vi "NMR14.vi"() -> ()   [LabVIEW 2013]
uses:
  <vilib>/Utility/file.llb/Read From Spreadsheet File (DBL).vi
  <vilib>/Analysis/NI_AALBase.lvlib
panel:
  in  "Q curve file":string="realback213.txt"
  out "File name 2":string="C:\\users\\plm\\Desktop\\rssmt\\realback213.txt"
  in  "AutoBaseline":bool
  out "RF OK":bool=TRUE
  out "Peak area (V-MHz)":sgl=3.3948524 format="%.3f"
  in  "Gauss Fit":bool
  out "NMR Graph + Fit":cluster{cluster{dbl, "Numeric":dbl}[]}[](graph)=[{[{212.6, "Numeric"=6.179833984375}, {212.608, "Numeric"=5.96031494140625}, {212.61599999999999, "Numeric"=5.74044189453125}, {212.624, "Numeric"=5.5264892578125}, {212.632, "Numeric"=5.31328125}, {212.64, "Numeric"=5.10472412109375}, {212.648, "Numeric"=4.900927734375}, {212.656, "Numeric"=4.704541015625}, {212.664, "Numeric"=4.511669921875}, {212.672, "Numeric"=4.3124755859375}, {212.68, "Numeric"=4.1198974609375}, {212.688, "Numeric"=3.935693359375}, {212.696, "Numeric"=3.76107177734375}, {212.704, "Numeric"=3.5800537109375}, {212.712, "Numeric"=3.40418701171875}, {212.72, "Numeric"=3.2398681640625}, {212.728, "Numeric"=3.0807373046875}, {212.736, "Numeric"=2.91600341796875}, {212.744, "Numeric"=2.76717529296875}, {212.752, "Numeric"=2.60875244140625}, {212.76, "Numeric"=2.45557861328125}, {212.768, "Numeric"=2.3186279296875}, {212.776, "Numeric"=2.17218017578125}, {212.784, "Numeric"=2.04324951171875}, {212.792, "Numeric"=1.9197265625}, {212.79999999999998, "Numeric"=1.78963623046875}, {212.808, "Numeric"=1.67039794921875}, {212.816, "Numeric"=1.54791259765625}, {212.82399999999998, "Numeric"=1.44422607421875}, {212.832, "Numeric"=1.32734375}, {212.84, "Numeric"=1.22919921875}, {212.84799999999998, "Numeric"=1.13302001953125}, {212.856, "Numeric"=1.03822021484375}, {212.864, "Numeric"=0.9540771484375}, {212.87199999999999, "Numeric"=0.87376708984375}, {212.88, "Numeric"=0.78779296875}, {212.888, "Numeric"=0.71485595703125}, {212.896, "Numeric"=0.63963623046875}, {212.904, "Numeric"=0.59088134765625}, {212.912, "Numeric"=0.532666015625}, {212.92, "Numeric"=0.4708251953125}, {212.928, "Numeric"=0.423828125}, {212.936, "Numeric"=0.37716064453125}, {212.944, "Numeric"=0.3446533203125}, {212.952, "Numeric"=0.32086181640625}, {212.96, "Numeric"=0.2843017578125}, {212.968, "Numeric"=0.270751953125}, {212.976, "Numeric"=0.2579833984375}, {212.984, "Numeric"=0.23699951171875}, {212.992, "Numeric"=0.23897705078125}, {213.0, "Numeric"=0.238916015625}, {213.008, "Numeric"=0.248974609375}, {213.016, "Numeric"=0.265283203125}, {213.024, "Numeric"=0.28079833984375}, {213.032, "Numeric"=0.300244140625}, {213.04, "Numeric"=0.33636474609375}, {213.048, "Numeric"=0.372314453125}, {213.056, "Numeric"=0.4180908203125}, {213.064, "Numeric"=0.4687255859375}, {213.072, "Numeric"=0.525830078125}, {213.08, "Numeric"=0.58543701171875}, {213.088, "Numeric"=0.6470947265625}, {213.096, "Numeric"=0.7219970703125}, {213.104, "Numeric"=0.81129150390625}, {213.112, "Numeric"=0.90042724609375}, {213.12, "Numeric"=0.9976318359375}, {213.12800000000001, "Numeric"=1.0961669921875}, {213.136, "Numeric"=1.19154052734375}, {213.144, "Numeric"=1.30576171875}, {213.15200000000002, "Numeric"=1.42882080078125}, {213.16, "Numeric"=1.55714111328125}, {213.168, "Numeric"=1.69908447265625}, {213.17600000000002, "Numeric"=1.83853759765625}, {213.184, "Numeric"=1.98814697265625}, {213.192, "Numeric"=2.1465087890625}, {213.2, "Numeric"=2.30396728515625}, {213.208, "Numeric"=2.4755859375}, {213.216, "Numeric"=2.64779052734375}, {213.224, "Numeric"=2.8399658203125}, {213.232, "Numeric"=3.03016357421875}, {213.24, "Numeric"=3.2257568359375}, {213.248, "Numeric"=3.4392822265625}, {213.256, "Numeric"=3.6543701171875}, {213.264, "Numeric"=3.87130126953125}, {213.272, "Numeric"=4.10189208984375}, {213.28, "Numeric"=4.33153076171875}, {213.288, "Numeric"=4.5672119140625}, {213.296, "Numeric"=4.82923583984375}, {213.304, "Numeric"=5.08277587890625}, {213.312, "Numeric"=5.3467041015625}, {213.32, "Numeric"=5.62410888671875}, {213.328, "Numeric"=5.90218505859375}, {213.336, "Numeric"=6.19228515625}, {213.344, "Numeric"=6.49820556640625}, {213.352, "Numeric"=6.7964599609375}, {213.36, "Numeric"=7.11771240234375}, {213.368, "Numeric"=7.44090576171875}, {213.376, "Numeric"=7.7695068359375}, {213.38400000000001, "Numeric"=8.12364501953125}, {213.392, "Numeric"=8.476611328125}, {213.4, "Numeric"=8.8313720703125}]}]
  in  "Amp of Q curve":dbl=1.7999999999999998 min=0.0 max=3.0 step=0.01 format="%_3f"
  in  "Subtract Q curve":bool
  in  "Adjust Tune":bool
  out "IF Offset":dbl(graph)=1.8102946533203148
  out "Pedestal Difference":dbl(graph)=1.261193033854167
  out "# Good Spectra":i32=1
  in  "Quality cuts":bool=TRUE
  out "Pedestal OK":bool
  out "Sweep #":i32=100
  out "1st Sweep":bool
  out "ADC volts OK":bool=TRUE
  out "Peak Height Distribution":cluster{"Y":dbl[], "Y":dbl[]}[](graph)=[{"Y"=[-99.0, -99.0, -99.0, -99.0, -99.0, -99.0, -99.0, -99.0, -99.0, -99.0, -99.0, -99.0, -99.0, -99.0, -99.0, -99.0, -99.0, -99.0, -99.0, -99.0, -99.0, -99.0, -99.0, -99.0, -99.0, -99.0, -99.0, -99.0, -99.0, -99.0, -99.0, -99.0, -99.0, -99.0, -99.0, -99.0, -99.0, -99.0, -99.0, -99.0, -99.0, -99.0, -99.0, -99.0, -99.0, -99.0, -99.0, -99.0, -99.0, -99.0, -99.0, -99.0, -99.0, -99.0, -99.0, -99.0, -99.0, -99.0, -99.0, -99.0, -99.0, -99.0, -99.0, -99.0, -99.0, -99.0, -99.0, -99.0, -99.0, -99.0, -99.0, -99.0, -99.0, -99.0, -99.0, -99.0, -99.0, -99.0, -99.0, -99.0, -99.0, -99.0, -99.0, -99.0, -99.0, -99.0, -99.0, -99.0, -99.0, -99.0, -99.0, -99.0, -99.0, -99.0, -99.0, -99.0, -99.0, -99.0, -99.0, -99.0], "Y"=[0.0, 0.0, 0.0, 0.0, 0.0, 0.0, 0.0, 0.0, 0.0, 0.0, 0.0, 0.0, 0.0, 0.0, 0.0, 0.0, 0.0, 0.0, 0.0, 0.0, 0.0, 0.0, 0.0, 0.0, 0.0, 0.0, 0.0, 0.0, 0.0, 0.0, 0.0, 0.0, 0.0, 0.0, 0.0, 0.0, 0.0, 0.0, 0.0, 0.0, 0.0, 0.0, 0.0, 0.0, 0.0, 0.0, 0.0, 0.0, 0.0, 0.0, 0.0, 0.0, 0.0, 0.0, 0.0, 0.0, 0.0, 0.0, 0.0, 0.0, 0.0, 0.0, 0.0, 0.0, 0.0, 0.0, 0.0, 0.0, 0.0, 0.0, 0.0, 0.0, 0.0, 0.0, 0.0, 0.0, 0.0, 0.0, 0.0, 0.0, 0.0, 0.0, 0.0, 0.0, 0.0, 0.0, 0.0, 0.0, 0.0, 0.0, 0.0, 0.0, 0.0, 0.0, 0.0, 0.0, 0.0, 0.0, 0.0, 1.0]}]
  in  "# of Sweeps":i32=100
  out "Std Dev (V)":dbl=nan format="%_2g"
  out "Peak mean (V)":dbl=-99.0 format="%_4g"
  out "Peak Height":dbl(graph)=8.8313720703125
  in  "Raw Data":bool=TRUE
  in  "Tank RF ON":bool=TRUE
  in  "IF Atten (dB)":i8 min=0 max=35 step=5
  in  "IFoffset (V)":dbl=1.8102946533203148 min=0.0 max=3000.0 step=0.001 format="%.3f"
  in  "Tune  (V)":dbl=1.6310000000000064 min=0.0 max=5.0 step=0.001 format="%.3f"
  in  "Hi / Lo Gain":bool
  out "Voltage Array":sgl[](array[numeric])=[6.179834, 5.9603148, 5.740442, 5.5264893, 5.313281, 5.104724, 4.9009275, 4.704541, 4.51167, 4.3124757, 4.1198974, 3.9356933, 3.7610717, 3.5800538, 3.404187, 3.2398682, 3.0807374, 2.9160035, 2.7671752, 2.6087525, 2.4555786, 2.3186278, 2.1721802, 2.0432496, 1.9197266, 1.7896363, 1.670398, 1.5479126, 1.444226, 1.3273437, 1.2291992, 1.13302, 1.0382202, 0.9540771, 0.8737671, 0.787793, 0.71485597, 0.6396362, 0.59088135, 0.532666, 0.4708252, 0.42382812, 0.37716064, 0.3446533, 0.32086182, 0.28430176, 0.27075195, 0.2579834, 0.23699951, 0.23897704, 0.23891601, 0.2489746, 0.2652832, 0.28079835, 0.30024415, 0.33636475, 0.37231445, 0.41809082, 0.4687256, 0.5258301, 0.585437, 0.6470947, 0.7219971, 0.8112915, 0.9004272, 0.99763185, 1.096167, 1.1915405, 1.3057617, 1.4288208, 1.5571411, 1.6990845, 1.8385376, 1.988147, 2.1465087, 2.3039672, 2.475586, 2.6477904, 2.8399658, 3.0301635, 3.225757, 3.4392822, 3.65437, 3.8713012, 4.101892, 4.3315306, 4.567212, 4.829236, 5.082776, 5.346704, 5.624109, 5.902185, 6.192285, 6.4982057, 6.79646, 7.1177125, 7.4409056, 7.769507, 8.123645, 8.476611, 8.831372] format="%.4f"
  in  "Invert Polarity":bool=TRUE
  out "Pedestal Diff (V)":sgl=1.261193 format="%.3f"
  out "Peak amp (V)":sgl=8.831372 format="%.3f"
  in  "Save Data to File":bool=TRUE
  in  "RF Level (dBm)":dbl=-1.0 min=-10.0 max=1.0 step=0.1 format="%.2f"
  out "SMT error out":errorcluster
  out "Sample RMS (V)":dbl=0.008836833866740928 format="%.4f"
  in  "# Sample/step":i32=100 min=1 max=1000 step=100
  in  "ADC Rate (Hz)":i32=10000 min=1 max=20000 step=1000
  in  "ADC Range":i32(ring)=1 items=["+- 10 V"=1, "+- 2.5 V"=3]
  in  "Step Width (MHz)":dbl=0.008 min=0.0 max=1000.0 step=0.0005 format="%.4f"
  in  "Freq Span (MHz)":dbl=0.8 min=0.0 max=3000.0 step=0.1 format="%.3f"
  in  "Center Freq (MHz)":dbl=213.0 min=0.005 max=6000.0 step=0.1 format="%.3f"
  in  "Sweep Mode":u16(ring)=3 items=["Off", "Single", "Auto", "Step"]
  in  "GPIB Addr (28)":refnum<visa-resource-name>="GPIB0::28::INSTR"
  # "Settings"
  # "E1039 Prototype NMR Control Panel"
  # "D\nA\nC"
  # "R\nF\n\nG\ne\nn\ne\nr\na\nt\no\nr"
  # "A\nD\nC"
  # "D\na\nt\na"
  # "I\n/\nO"
  # "Results"
  # "A\nv\ne\nr\na\ng\ne"
  # "S\nw\ne\ne\np"
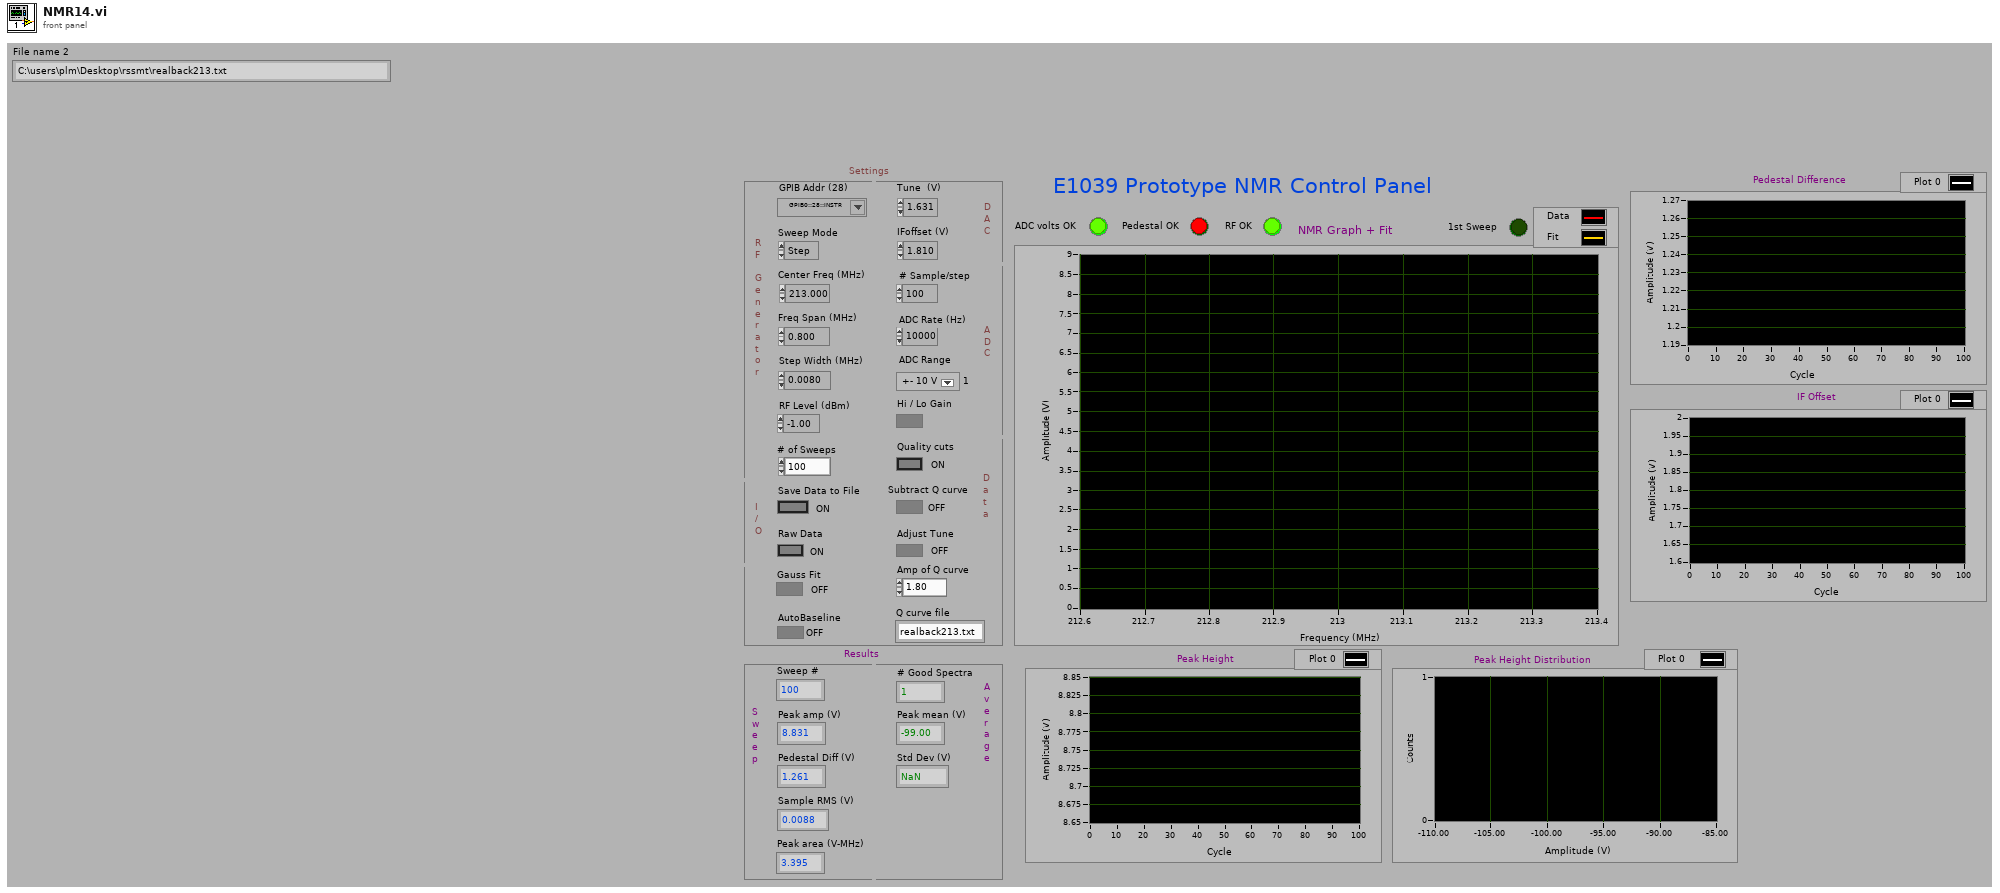
[diagram p1: front panel]
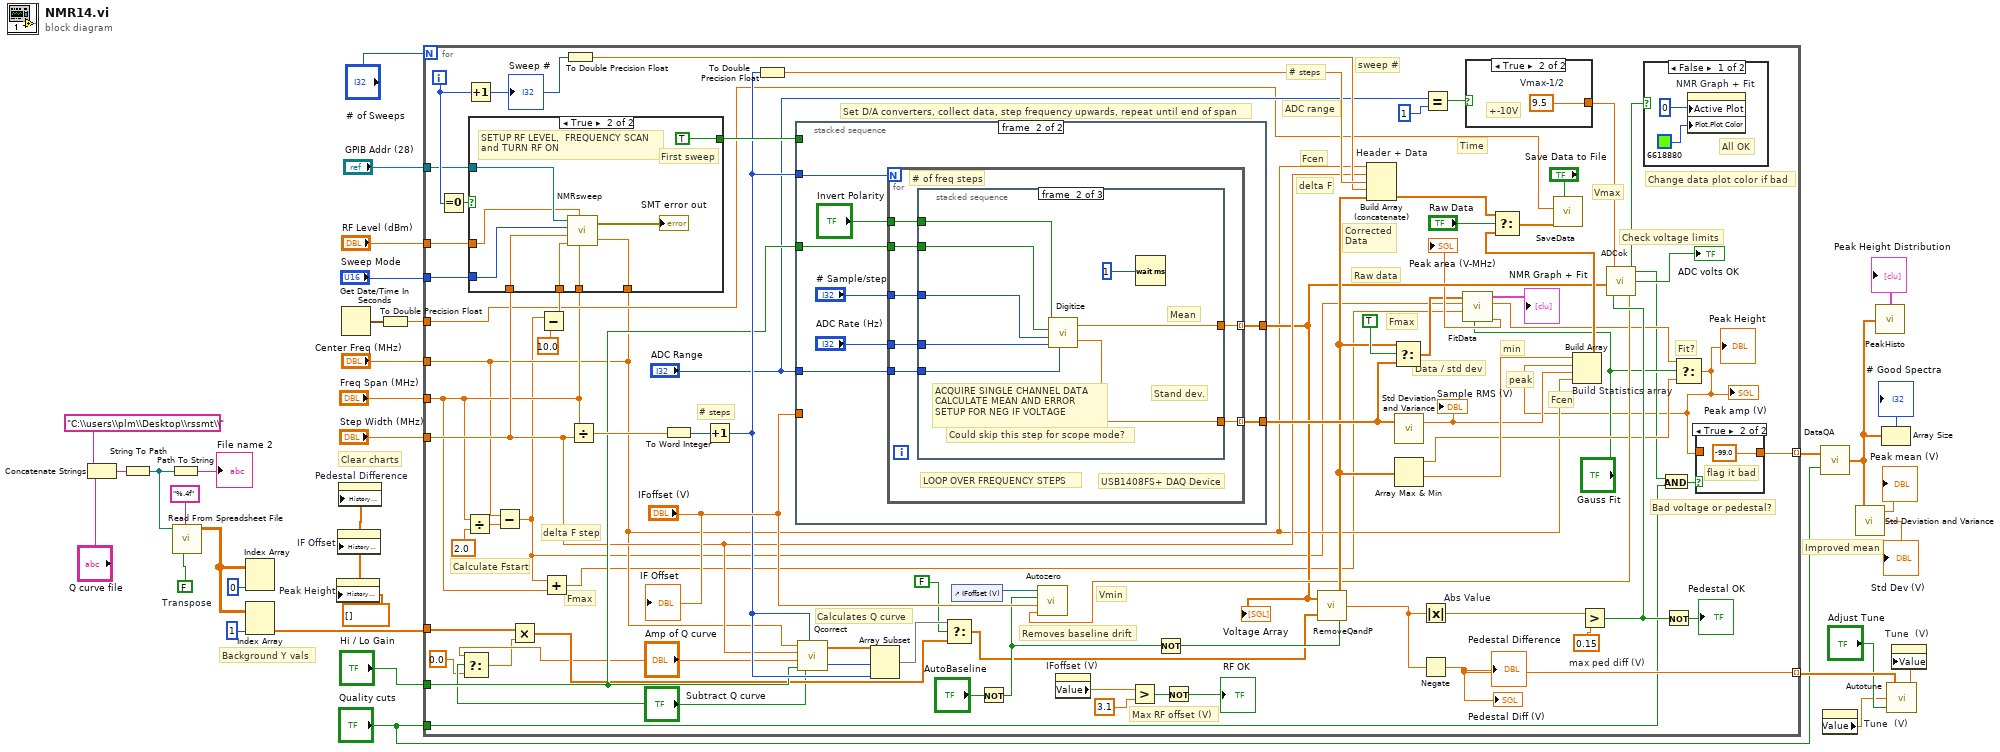
[diagram p0: block diagram]
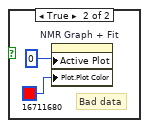
[diagram p2: hidden frame]
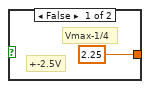
[diagram p3: hidden frame]
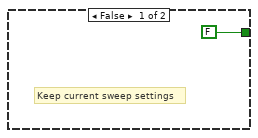
[diagram p5: hidden frame]
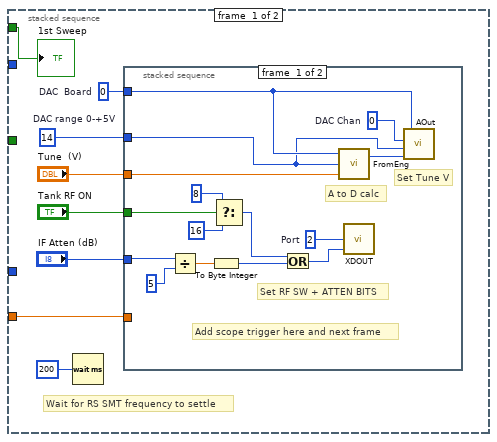
[diagram p6: hidden frame]
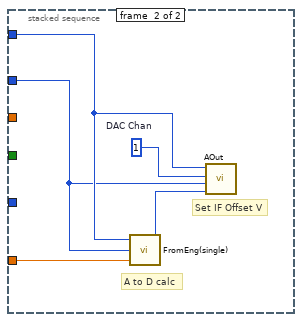
[diagram p7: hidden frame]
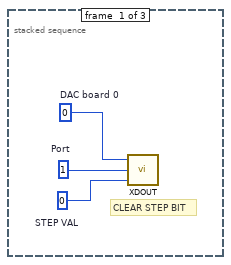
[diagram p8: hidden frame]
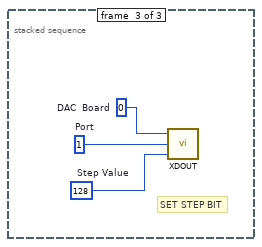
[diagram p9: hidden frame]
diagram:
  w8 = FALSE  # Transpose
  w17 = dbl[] []
  # "Background Y vals"
  # "Clear charts"
  # "Improved mean"
  n1 = Concatenate Strings "Concatenate Strings"("C:\\users\\plm\\Desktop\\rssmt\\", "Q curve file") -> (w11:string)
  n2 = String To Path(string=w11) -> (path=w7:path)
  n3 = Path To String(path=w7) -> (string=→"File name 2":string)
  n4 = call-poly <vilib>:"Read From Spreadsheet File.vi"("transpose (no:F)"=w8, "format (%.3f)"="%.4f", "file path (dialog if empty)"=w7) -> ("all rows"=w6:dbl[][])  [unwired: 4 in, 4 out]
  n5 = Index Array "Index Array"(array=w6, index (col)=0) -> ()  [unwired: 1 in, 1 out]
  n6 = Index Array(array=w6, index (col)=1) -> (element=w1:dbl[])  [unwired: 1 in]
  n7 = property on="Peak Height" class="WFChart (strict)"("History Data"=w17) -> ()  [unwired: 2 in, 2 out]
  n8 = property on="IF Offset" class="WFChart (strict)"("History Data"=w17) -> ()  [unwired: 2 in, 2 out]
  n9 = property on="Pedestal Difference" class="WFChart (strict)"("History Data"=w17) -> ()  [unwired: 2 in, 2 out]
  n10 = Get Date/Time In Seconds() -> (seconds since 1Jan1904=w13:timestamp)
  n11 = To Double Precision Float(number=w13) -> (double precision float=w12:dbl)
  n12 = for {
    N: "# of Sweeps" -> [_]
    tunnel: [w94] -> w29 mode=indexing
    tunnel: "Quality cuts" -> [w68]
    tunnel: [w77] -> w26 mode=indexing
    tunnel: "Center Freq (MHz)" -> [w55]
    tunnel: "Freq Span (MHz)" -> [w61]
    tunnel: "Step Width (MHz)" -> [w67]
    tunnel: "Sweep Mode" -> [w81]
    tunnel: "Hi / Lo Gain" -> [w80]
    tunnel: "GPIB Addr (28)" -> [w79]
    tunnel: "RF Level (dBm)" -> [w78]
    tunnel: w12 -> [w62]
    tunnel: w1 -> [w39]
    i -> [w92]
    w95 = 0.15  # max ped diff (V)
    # "Vmax"
    # "Change data plot color if bad"
    # "Max RF offset (V)"
    # "Fmax"
    # "Fit?"
    # "Fmax"
    # "Time"
    # "Vmin"
    # "min"
    # "peak"
    # "Raw data"
    # "Corrected\nData"
    # "Fcen"
    # "delta F"
    # "# steps"
    # "ADC range"
    # "sweep #"
    # "Fcen"
    # "Set D/A converters, collect data, step frequency upwards, repeat until end of span"
    # "Calculates Q curve"
    # "Removes baseline drift"
    # "Bad voltage or pedestal?"
    # "Check voltage limits"
    # "Data / std dev"
    # "# steps"
    # "Calculate Fstart"
    # "delta F step"
    n13 = Equal To 0?(x=w92) -> (x = 0?=w97:bool)
    n14 = Select(t="Amp of Q curve", s="Subtract Q curve", f=0.0) -> (s? t:f=w34:dbl)
    n15 = Divide(x=w61, y=sgl 2.0) -> (x/y=w108:dbl)
    n16 = Increment(x=w92) -> (x+1=w82:i32)
    "Sweep #" <- w82
    n17 = Subtract(x=w55, y=w108) -> (x-y=w50:dbl)
    n18 = Multiply(x=w39, y=w34) -> (x*y=w38:dbl[])
    n19 = Subtract(x=w50, y=10.0) -> (x-y=w106:dbl)
    n20 = case shown="True" w97 {
      tunnel: w106 -> [_ w128]
      tunnel: w67 -> [_ w126]
      tunnel: w55 -> [_ w125]
      tunnel: w61 -> [_ w127]
      tunnel: [FALSE TRUE] -> w96
      tunnel: w81 -> [_ w122]
      tunnel: w79 -> [_ w121]
      tunnel: w78 -> [_ w120]
      frame False {
        # "Keep current sweep settings"
      }
      frame True {
        # "First sweep"
        # "SETUP RF LEVEL,  FREQUENCY SCAN\nand TURN RF ON"
        n21 = call "NMRsweep.vi"("Center Freq (MHz)"=w125, "Freq Span (MHz)"=w127, "RF Level (dBm)"=w120, "Foffset (MHz)"=w128, "Step Width (MHz)"=w126, "Sweep Mode"=w122, "GPIB Addr (28)"=w121) -> ("error out"=→"SMT error out":errorcluster)
      }
    }
    n22 = Add(x=w50, y=w61) -> (x+y=w49:dbl)
    n23 = To Double Precision Float(number=w82) -> (double precision float=w83:dbl)
    n24 = Divide(x=w61, y=w67) -> (x/y=w110:dbl)
    n25 = To Word Integer(number=w110) -> (16bit integer=w107:i16)
    n26 = Increment(x=w107) -> (x+1=w86:i16)
    n27 = To Double Precision Float(number=w86) -> (double precision float=w85:dbl)
    n28 = stacked-sequence {
      tunnel: [_ w164] -> w100
      tunnel: [_ w163] -> w65
      tunnel: w86 -> [_ w162]
      tunnel: "IFoffset (V)" -> [w130 _]
      tunnel: w80 -> [_ w161]
      tunnel: w96 -> [w129 _]
      tunnel: "ADC Range" -> [_ w160]
      frame #0 {
        w134 = 14  # DAC range 0-+5V
        w135 = 0  # DAC  Board
        # "Wait for RS SMT frequency to settle"
        n29 = Wait (ms)(milliseconds to wait=200) -> ()  [unwired: 1 out]
        n30 = stacked-sequence {
          tunnel: w135 -> [w142 w154]
          tunnel: w134 -> [w141 w153]
          tunnel: "Tune  (V)" -> [w140 _]
          tunnel: "Tank RF ON" -> [w138 _]
          tunnel: "IF Atten (dB)" -> [w137 _]
          tunnel: w130 -> [_ w152]
          frame #0 {
            w144 = 2  # Port
            w151 = 0  # DAC Chan
            # "Add scope trigger here and next frame"
            # "A to D calc"
            # "Set RF SW + ATTEN BITS"
            # "Set Tune V"
            n31 = Divide(x=w137, y=5) -> (x/y=w149:dbl)
            n32 = To Byte Integer(number=w149) -> (8bit integer=w146:i8)
            n33 = Select(t=8, s=w138, f=16) -> (s? t:f=w145:i32)
            n34 = Or(x=w145, y=w146) -> (x .or. y?=w143:i32)
            n35 = call-poly "FromEng.VI"("Eng Units"=w140, "Range"=w141, "BoardNum (0)"=w142) -> ("DA Data"=w139:u16)  [unwired: 1 out]
            n36 = call "XDOUT.VI"(2:w143, "PortNum"=w144) -> ()  [unwired: 3 in]
            n37 = call "AOut.VI"("DataValue"=w139, "Range"=w141, "Channel"=w151, "BoardNum"=w142) -> ()  [unwired: 1 out]
          }
          frame #1 {
            w156 = 1  # DAC Chan
            # "A to D calc"
            # "Set IF Offset V"
            n38 = call "FromEng(single).VI"("Eng Units"=w152, "Range"=w153, "BoardNum (0)"=w154) -> ("DA Data"=w155:u16)  [unwired: 1 out]
            n39 = call "AOut.VI"("DataValue"=w155, "Range"=w153, "Channel"=w156, "BoardNum"=w154) -> ()  [unwired: 1 out]
          }
        }
        "1st Sweep" <- w129
      }
      frame #1 {
        n40 = for {
          N: w162 -> [_]
          tunnel: [w171] -> w163 mode=indexing
          tunnel: [w170] -> w164 mode=indexing
          tunnel: w161 -> [w169]
          tunnel: w160 -> [w168]
          tunnel: "ADC Rate (Hz)" -> [w167]
          tunnel: "# Sample/step" -> [w166]
          tunnel: "Invert Polarity" -> [w165]
          # "# of freq steps"
          # "USB1408FS+ DAQ Device"
          # "LOOP OVER FREQUENCY STEPS"
          n41 = stacked-sequence {
            tunnel: [_ w181 _] -> w171
            tunnel: [_ w180 _] -> w170
            tunnel: w169 -> [_ w179 _]
            tunnel: w168 -> [_ w178 _]
            tunnel: w167 -> [_ w177 _]
            tunnel: w166 -> [_ w176 _]
            tunnel: w165 -> [_ w175 _]
            frame #0 {
              w172 = 0  # DAC board 0
              w173 = 0  # STEP VAL
              w174 = 1  # Port
              # "CLEAR STEP BIT"
              n42 = call "XDOUT.VI"(2:w173, "PortNum"=w174, "BoardNum"=w172) -> ()  [unwired: 2 in]
            }
            frame #1 {
              # "Could skip this step for scope mode?"
              # "Stand dev."
              # "Mean"
              # "ACQUIRE SINGLE CHANNEL DATA\nCALCULATE MEAN AND ERROR\nSETUP FOR NEG IF VOLTAGE"
              n43 = call "Digitize.vi"("Invert Polarity"=w175, "IF or Log"=w179, "# Sample/step"=w176, "ADC Rate (Hz)"=w177, "ADC Range"=w178) -> ("mean"=w181:dbl, "standard deviation"=w180:dbl)
              n44 = Wait (ms)(milliseconds to wait=1) -> ()  [unwired: 1 out]
            }
            frame #2 {
              w183 = 128  # Step Value
              w185 = 0  # DAC  Board
              w184 = 1  # Port
              # "SET STEP BIT"
              n45 = call "XDOUT.VI"(2:w183, "PortNum"=w184, "BoardNum"=w185) -> ()  [unwired: 2 in]
            }
          }
        }
      }
    }
    "Voltage Array" <- w65
    n46 = call "Qcorrect.vi"("Subtract Q curve"="Subtract Q curve", "Nstep"=w86, "IF or Log"=w80, "Amp of Q curve"="Amp of Q curve", "Step Width (MHz)"=w67, "Center Freq (MHz)"=w55) -> ("Start"=w101:i32, "Array"=w102:dbl[])
    n47 = Array Subset "Array Subset"(array=w102, index=w101, length=w86) -> (w42:dbl[])
    n48 = Select(t=w42, s=FALSE, f=w38) -> (s? t:f=w41:dbl[])
    n49 = control-ref of="IFoffset (V)"() -> (w71:refnum<vi>)
    n50 = Not(x="AutoBaseline") -> (.not. x?=w44:bool)
    n51 = property on="IFoffset (V)" class="DigNum (strict)"() -> ("Value"=w59:dbl)  [unwired: 2 in, 2 out]
    n52 = Greater?(x=w59, y=3.1) -> (0:w57:bool)
    n53 = Not(x=w44) -> (.not. x?=w43:bool)
    n54 = Not(x=w57) -> (.not. x?=→"RF OK":bool)
    n55 = call "RemoveQandP.vi"("Raw data"=w65, "Qcurve"=w41, "Subtract Ped?"=w43) -> ("Corrected data"=w84:dbl[], "Ped L-R"=w88:dbl)
    n56 = Build Array (concatenate) "Header + Data"(w55, w67, w85, w83, w84) -> (w87:dbl[])
    n57 = Select(t=w84, s=TRUE, f=w100) -> (s? t:f=w51:dbl[])
    n58 = call <vilib>:"Std Deviation and Variance.vi"("X"=w100) -> ("mean"=w66:dbl)  [unwired: 1 in, 2 out]
    "Sample RMS (V)" <- w66
    n59 = Array Max & Min(array=w84) -> (max value=w60:dbl, min value=w99:dbl)  [unwired: 2 out]
    n60 = Absolute Value "Abs Value"(x=w88) -> (abs(x)=w90:dbl)
    n61 = Negate(x=w88) -> (-x=w77:dbl)
    "Pedestal Diff (V)" <- w77
    "Pedestal Difference" <- w77
    n62 = Equal?(x="ADC Range", y=1) -> (x = y?=w75:bool)
    n63 = call "FitData.vi"("Fit?"="Gauss Fit", "Fmax"=w49, "Fmin"=w50, "Yarray"=w51) -> ("Peak Area (V-MHz)"=→"Peak area (V-MHz)":dbl, "Amplitude (V)"=w53:dbl, "NMR Graph + Fit"=→"NMR Graph + Fit":cluster{cluster{dbl, "Numeric":dbl}[]}[])  [unwired: 2 out]
    n64 = case shown="True" w75 {
      tunnel: [2.25 w116] -> w72
      frame False {
        # "Vmax-1/4"
        # "+-2.5V"
      }
      frame True {
        w116 = 9.5  # Vmax-1/2
        # "+-10V"
      }
    }
    n65 = Greater?(x=w90, y=w95) -> (0:w76:bool)
    n66 = call "ADCok.vi"("PedOK"=w76, "Array"=w65, "Vmax-1/2"=w72) -> ("Vmin"=w70:dbl, "ADC voltages OK"=→"ADC volts OK":bool, "Allok"=w47:bool)
    n67 = call "Autozero.vi"("Vmin (V)"=w70, "IFoffset (V)"="IFoffset (V)", "IF or Log"=w44, "reference"=w71) -> ()
    n68 = case shown="False" w47 {
      frame False {
        # "All OK"
        n69 = property on="NMR Graph + Fit" class="XYGraph (strict)"("Active Plot"=0, "Plot.Plot Color"=u32 6618880) -> ()  [unwired: 2 in, 2 out]
      }
      frame True {
        # "Bad data"
        n70 = property on="NMR Graph + Fit" class="XYGraph (strict)"("Active Plot"=0, "Plot.Plot Color"=u32 16711680) -> ()  [unwired: 2 in, 2 out]
      }
    }
    n71 = And(x=w47, y=w68) -> (x .and. y?=w91:bool)
    n72 = Not(x=w76) -> (.not. x?=→"Pedestal OK":bool)
    n73 = Select(t=w53, s="Gauss Fit", f=w60) -> (s? t:f=w46:dbl)
    "Peak amp (V)" <- w46
    "Peak Height" <- w46
    n74 = Build Array "Build Statistics array"(w99, w46, w66, w55) -> (w105:dbl[])
    n75 = Select(t=w87, s="Raw Data", f=w105) -> (s? t:f=w63:dbl[])
    n76 = call "SaveData.vi"("Array"=w63, "Save Data to File"="Save Data to File", "Ext time (sec)"=w62) -> ()  [unwired: 1 out]
    n77 = case shown="True" w91 {
      tunnel: [w117 -99.0] -> w94
      tunnel: w46 -> [w117 _]
      frame False {
        # "Data OK"
      }
      frame True {
        # "flag it bad"
      }
    }
    "IF Offset" <- "IFoffset (V)"
  }
  n78 = call "DataQA.vi"("Quality cuts"="Quality cuts", "Data In"=w29) -> ("Data Out"=w28:dbl[])
  n79 = property on="Tune  (V)" class="DigNum (strict)"() -> ("Value"=w16:dbl)  [unwired: 2 in, 2 out]
  n80 = call <vilib>:"Std Deviation and Variance.vi"("X"=w28) -> ("mean"=→"Peak mean (V)":dbl, "standard deviation"=→"Std Dev (V)":dbl)  [unwired: 1 in, 1 out]
  n81 = call "PeakHisto.vi"("Data Out"=w28) -> ("XY Graph"=→"Peak Height Distribution":cluster{"Y":dbl[], "Y":dbl[]}[])
  n82 = Array Size(array=w28) -> (size(s)=→"# Good Spectra":i32)
  n83 = call "Autotune.vi"("Adjust Tune"="Adjust Tune", "Tune Vin"=w16, "Pedestal Diff"=w26) -> ("Tune Vout"=w15:dbl)
  n84 = property on="Tune  (V)" class="DigNum (strict)"("Value"=w15) -> ()  [unwired: 2 in, 2 out]
